vi "DAQ_send_digital_pulse.vi"(3 "error in":errorcluster, 4 "Pulse length (ms)":u32=250, 5 "Digital input":tag) -> (0 "error out":errorcluster)   [LabVIEW 2015]
uses:
  <vilib>/DAQmx/write.llb/DAQmx Write (Digital Bool 1Line 1Point).vi
  <vilib>/DAQmx/create/channels.llb/DAQmx Create Channel (DO-Digital Output).vi
  <vilib>/DAQmx/miscellaneous.llb/DAQmx Fill In Error Info.vi
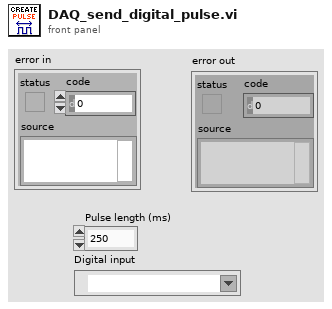
[diagram p1: front panel]
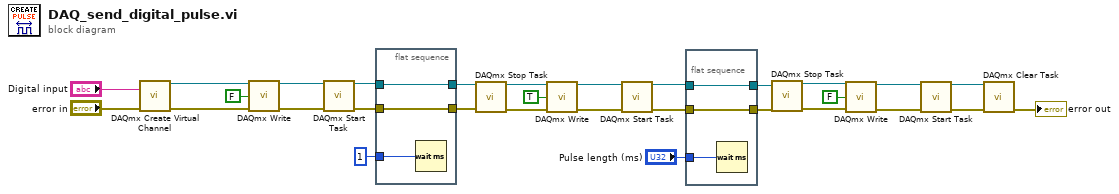
[diagram p0: block diagram]
diagram:
  n1 = call-poly <vilib>:"DAQmx Create Virtual Channel.vi"("lines"="Digital input", "error in"="error in") -> ("task out"=w13:refnum<k21>, "error out"=w12:errorcluster)  [unwired: 12 in]
  n2 = call-poly <vilib>:"DAQmx Write.vi"("task/channels in"=w13, "data"=FALSE, "error in"=w12) -> ("task out"=w15:refnum<k21>, "error out"=w16:errorcluster)  [unwired: 10 in, 1 out]
  n3 = call <vilib>:"DAQmx Start Task.vi"("task/channels in"=w15, "error in"=w16) -> ("task out"=w18:refnum<k21>, "error out"=w17:errorcluster)  [unwired: 12 in]
  n4 = flat-sequence {
    tunnel: w17 -> [w33]
    tunnel: w18 -> [w32]
    tunnel: [w33] -> w9
    tunnel: [w32] -> w10
    tunnel: u32 1 -> [w31]
    frame #0 {
      n5 = Wait (ms)(milliseconds to wait=w31) -> ()  [unwired: 1 out]
    }
  }
  n6 = call <vilib>:"DAQmx Stop Task.vi"("task/channels in"=w10, "error in"=w9) -> ("task out"=w7:refnum<k21>, "error out"=w8:errorcluster)  [unwired: 12 in]
  n7 = call-poly <vilib>:"DAQmx Write.vi"("task/channels in"=w7, "data"=TRUE, "error in"=w8) -> ("task out"=w28:refnum<k21>, "error out"=w27:errorcluster)  [unwired: 10 in, 1 out]
  n8 = call <vilib>:"DAQmx Start Task.vi"("task/channels in"=w28, "error in"=w27) -> ("task out"=w25:refnum<k21>, "error out"=w26:errorcluster)  [unwired: 12 in]
  n9 = flat-sequence {
    tunnel: w26 -> [w36]
    tunnel: w25 -> [w35]
    tunnel: [w36] -> w5
    tunnel: [w35] -> w6
    tunnel: "Pulse length (ms)" -> [w34]
    frame #0 {
      n10 = Wait (ms)(milliseconds to wait=w34) -> ()  [unwired: 1 out]
    }
  }
  n11 = call <vilib>:"DAQmx Stop Task.vi"("task/channels in"=w6, "error in"=w5) -> ("task out"=w4:refnum<k21>, "error out"=w3:errorcluster)  [unwired: 12 in]
  n12 = call-poly <vilib>:"DAQmx Write.vi"("task/channels in"=w4, "data"=FALSE, "error in"=w3) -> ("task out"=w23:refnum<k21>, "error out"=w24:errorcluster)  [unwired: 10 in, 1 out]
  n13 = call <vilib>:"DAQmx Start Task.vi"("task/channels in"=w23, "error in"=w24) -> ("task out"=w21:refnum<k21>, "error out"=w20:errorcluster)  [unwired: 12 in]
  n14 = call <vilib>:"DAQmx Clear Task.vi"("task in"=w21, "error in"=w20) -> ("error out"=→"error out":errorcluster)  [unwired: 13 in]
